vi "CRYSave Main Confiure.vi"   [LabVIEW 2013]
uses:
  CRYWindow/SubVI/CRYMain Sub Window Global.vi
panel:
  # "Save Main Configuration."
types:
  T1 = cluster{"Section":string, "Item":cluster{"Key":string, "Value":string}[]}
  T2 = enum32{"Invalid", "Standard", "Closed", "Hidden", "Minimized", "Maximized"}
  T3 = typedef "LVRectTypeDef.ctl" = cluster{"Left":i16, "Top":i16, "Right":i16, "Bottom":i16}
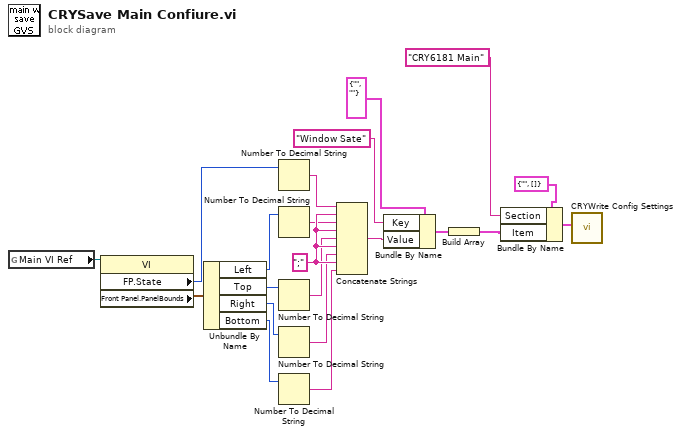
[diagram p0: block diagram]
diagram:
  w10 = ";" ("string")
  n1 = global read "CRYMain Sub Window Global.vi" "Main VI Ref"() -> (w21:refnum<vi>)
  n2 = property class="VI"(reference=w21) -> ("FP.State"=w13:T2, "Front Panel.PanelBounds"=w11:T3)  [unwired: 1 in, 2 out]
  n3 = Unbundle By Name(w11) -> ("Left"=w9:i16, "Top"=w8:i16, "Right"=w7:i16, "Bottom"=w6:i16)
  n4 = Number To Decimal String(number=w13) -> (decimal integer string=w12:string)  [unwired: 1 out]
  n5 = Number To Decimal String(number=w9) -> (decimal integer string=w5:string)  [unwired: 1 out]
  n6 = Number To Decimal String(number=w8) -> (decimal integer string=w4:string)  [unwired: 1 out]
  n7 = Number To Decimal String(number=w7) -> (decimal integer string=w3:string)  [unwired: 1 out]
  n8 = Number To Decimal String(number=w6) -> (decimal integer string=w2:string)  [unwired: 1 out]
  n9 = Concatenate Strings(w12, w10, w5, w10, w4, w10, w3, w10, w2) -> (w1:string)
  n10 = Bundle By Name(cluster=cluster{"Key":string, "Value":string} {"Key"="", "Value"=""} ("Cluster"), "Key"="Window Sate" ("Section"), "Value"=w1) -> (w16:cluster{"Key":string, "Value":string})
  n11 = Build Array(w16) -> (w15:cluster{"Key":string, "Value":string}[])
  n12 = Bundle By Name(cluster=T1 {"Section"="", "Item"=[]}, "Section"="CRY6181 Main", "Item"=w15) -> (w14:T1)
  n13 = call "CRYWrite Config Settings.vi"("Config Data"=w14) -> ()  [unwired: 1 in, 8 out]
